vi "Arduino Finite Analog Sampling.vi"() -> ()   [LabVIEW 2011, in "LabVIEW Interface for Arduino.lvlib"]
doc: "This example acquires a finite number of samples from an Analog Input."
uses:
  vi.lib/LabVIEW Interface for Arduino/LabVIEW Interface for Arduino.lvlib
panel:
  in  "VISA resource name":refnum<visa-resource-name>
  in  "Analog Input Pin":u8
  out "Data":waveform(dbl)(graph)
  in  "Acquition Speed (HZ)":u16=500
  in  "Number of Samples":u16
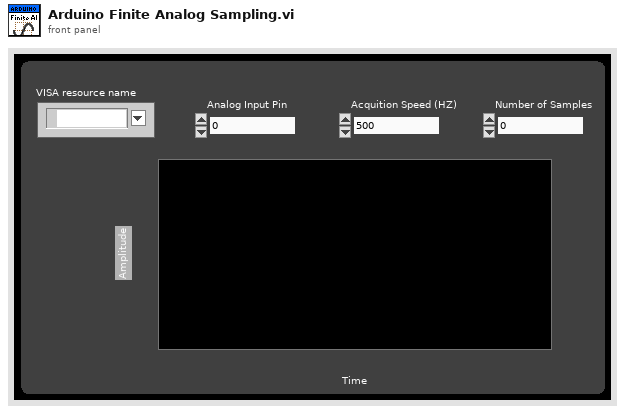
[diagram p1: front panel]
types:
  T1 = typedef "LabVIEW Interface for Arduino.lvlib/Arduino Resource.ctl" = cluster{"VISA resource":refnum<visa-resource-name>, "Board Type":T2, "Connection Type":enum8{"USB / Serial"}, "Bytes Per Packet (15)":u8}
  T2 = typedef "LabVIEW Interface for Arduino.lvlib/Board Type.ctl" = enum16{"Arduino Uno", "Dimuelanove w/Atmega 328", "Mega 2560", "Chipkit Uno32", "Chipkit Max32"}
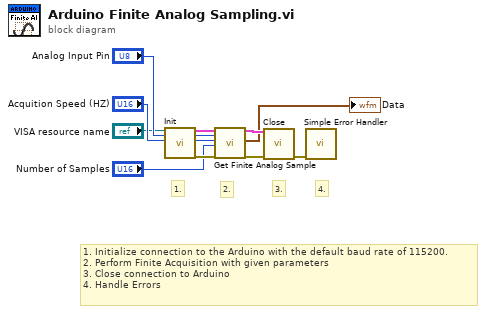
[diagram p0: block diagram]
diagram:
  # "4."
  # "3."
  # "2."
  # "1."
  # "1. Initialize connection to the Arduino with the default baud rate of 115200.\n2. Perform Finite Acquisition with given parameters\n3. Close connection to Arduino\n4. Handle Errors"
  n1 = call "Init.vi"("VISA resource"="VISA resource name") -> ("Arduino Resource"=w10:T1, "error out"=w6:errorcluster)  [unwired: 17 in]
  n2 = call "Get Finite Analog Sample.vi"("Arduino Resource"=w10, "Analog Input Pin"="Analog Input Pin", "Acquition Speed (HZ)"="Acquition Speed (HZ)", "Number of Samples"="Number of Samples", "error in"=w6) -> ("Arduino Resource"=w9:T1, "Data"=→"Data":waveform(dbl), "error out"=w7:errorcluster)  [unwired: 11 in, 1 out]
  n3 = call "Close.vi"("Arduino Resource"=w9, "error in"=w7) -> ("error out"=w8:errorcluster)  [unwired: 13 in]
  n4 = call <vilib>:"Simple Error Handler.vi"("error in (no error)"=w8) -> ()  [unwired: 4 in, 5 out]
